vi "UDP Data Link Global.vi"() -> ()   [LabVIEW 2015, in "UDP Data Link Shared.lvlib"]
uses:
  UDP Data Link Shared.lvlib
panel:
  in  "Rx Channel Destination Ref":string="Rx Channel Destination Ref"
  in  "Export File Location":string="Export File Location"
  in  "Export to File Status":string="Export to File Status"
  in  "Rx Channel Description":string="Rx Channel Description"
  in  "Rx Channel Destination Path":string="Rx Channel Destination Path"
  in  "Tx Remove Channel Button ID":string="NIVS_UDPDataLink_Tx_RemoveChannels"
  in  "Rx Channel Delete Indices":string="Rx Channel Delete Indices"
  in  "Tx Channel Delete Indices":string="Tx Channel Delete Indices"
  in  "Rx Channel Refs":string="Rx Channel Refs"
  in  "Tx Channel Refs":string="Tx Channel Refs"
  in  "Rx Channel Paths":string="Rx Channel Paths"
  in  "Rx Channel Names":string="Rx Channel Names"
  in  "Tx Channel Paths":string="Tx Channel Paths"
  in  "Tx Channel Names":string="Tx Channel Names"
  in  "Rx Channel Page GUID":string="63c7125a-181b-4c57-9d03-ed07a76e0610"
  in  "Tx Channels Section GUID":string="0bc41655-0fbd-46a2-8ece-b4a2475f5717"
  in  "Decimation":string="Decimation"
  in  "IP of Local NIC State":string="IP of Local NIC State"
  in  "Auto-Assign IP":string="Auto-Assign IP"
  in  "Rx Channels Section GUID":string="bf23c88a-fe1c-464c-adb1-d52dd120e94d"
  in  "Status Channels Section GUID":string="45116863-0d4e-47da-b92c-2c272c8a9276"
  in  "Status Channels GUID":string="d537c0a0-5451-4b3d-9770-fed708507db4"
  in  "TimeStamp Ref":string="TimeStamp Ref"
  in  "Server Port":string="Server Port"
  in  "IP of Remote NIC":string="IP of Remote NIC"
  in  "IP of Local NIC":string="IP of Local NIC"
  in  "Rx FIFO Timeout":string="Rx FIFO Timeout"
  in  "Rx FIFO Polling Rate":string="Rx FIFO Polling Rate"
  # "Main Page Properties"
  # "Rx Channels Section Properties"
  # "Tx Channels Section Properties"
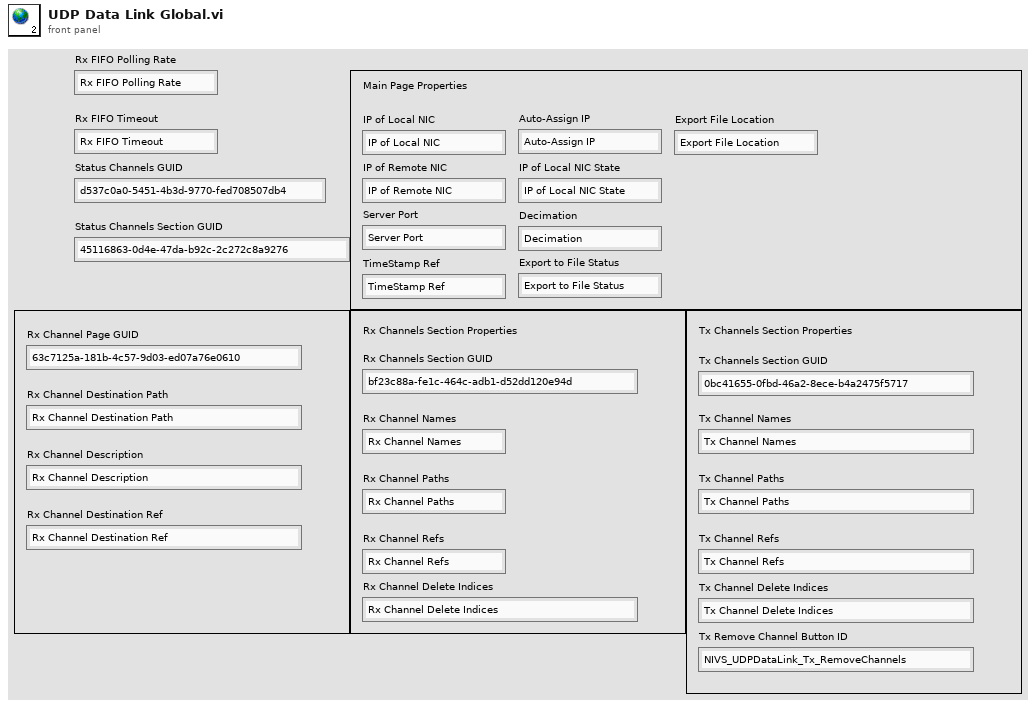
[diagram p1: front panel]
diagram:
